vi "Get Owner.vi"(8 "error in (no error)":errorcluster caption="错误输入（无错误）", 11 "Generic输入":refnum<class "Generic.lvclass">) -> (0 "error out":errorcluster caption="错误输出", 2 "Owner":refnum<data-value>, 3 "Generic输出":refnum<class "Generic.lvclass">)   [LabVIEW 2013, in "Hierarchy Framework.lvlib" / "Generic.lvclass"]
uses:
  Generic.lvclass
  Generic.lvclass/Generic.ctl
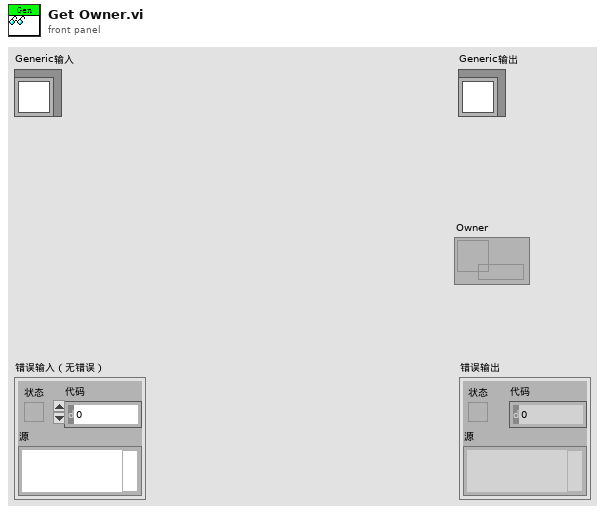
[diagram p1: front panel]
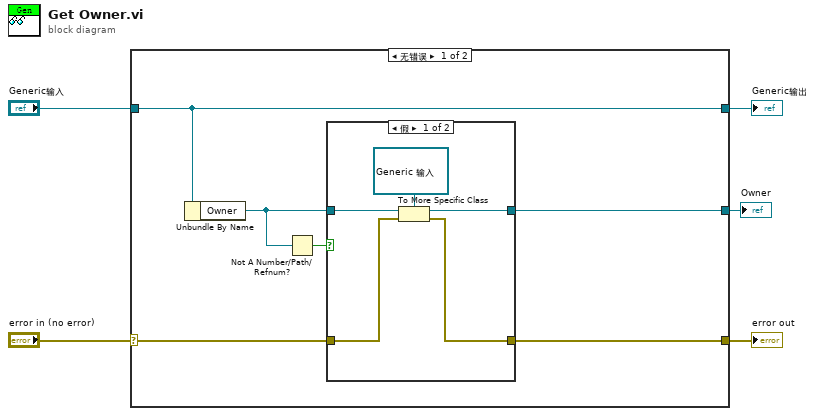
[diagram p0: block diagram]
diagram:
  n1 = case shown="无错误" "error in (no error)" {
    selector: "error in (no error)" -> [w9 w19]
    tunnel: [w8 w19] -> w4
    tunnel: [w11 w18] -> w2
    tunnel: "Generic输入" -> [w11 w18]
    tunnel: [w10 _] -> w1
    frame No Error {
      n2 = Unbundle By Name(w11) -> ("Owner"=w7:refnum<data-value>)
      n3 = Not A Number/Path/Refnum?(number/path/refnum=w7) -> (NaN/Path/Refnum?=w6:bool)
      n4 = case shown="假" w6 {
        tunnel: [w15 _] -> w10
        tunnel: w9 -> [w14 w17]
        tunnel: [w13 w17] -> w8
        tunnel: w7 -> [w12 _]
        frame False {
          n5 = To More Specific Class(target class=refnum<data-value> refnum ("数据值引用"), reference=w12, error in=w14) -> (specific class reference=w15:refnum<data-value>, error out=w13:errorcluster)
        }
        frame True {
        }
      }
    }
    frame Error {
    }
  }
  "error out" <- w4
  "Generic输出" <- w2
  "Owner" <- w1
